vi "Insert Front Panel.vi"(8 "error in (no error)":errorcluster, 9 "Insertion Request Time":timestamp, 10 "Protected Subpanel":T1, 11 "IViewable in":refnum<class "IViewable.lvclass">) -> (0 "error out":errorcluster, 3 "IViewable out":refnum<class "IViewable.lvclass">)   [LabVIEW 2015, in "IViewable.lvlib" / "IViewable.lvclass"]
doc: "<License>\nCopyright © 2017 Composed Systems, LLC | All rights reserved\nwww.composed.io\n\nAuthor: Ethan Stern <ethan.stern@composed.io>\n\nThis software is provided \"AS IS\" WITHOUT WARRANTIES, either express or implied, AND IS FOR EDUCATIONAL PURPOSES ONLY.\n</License>"
uses:
  IViewable.lvclass
  ProtectedSubpanel/Protected Subpanel Reference.ctl
  ProtectedSubpanel/ProtectedSubpanel.lvclass
  IViewable.lvclass/IViewable.ctl
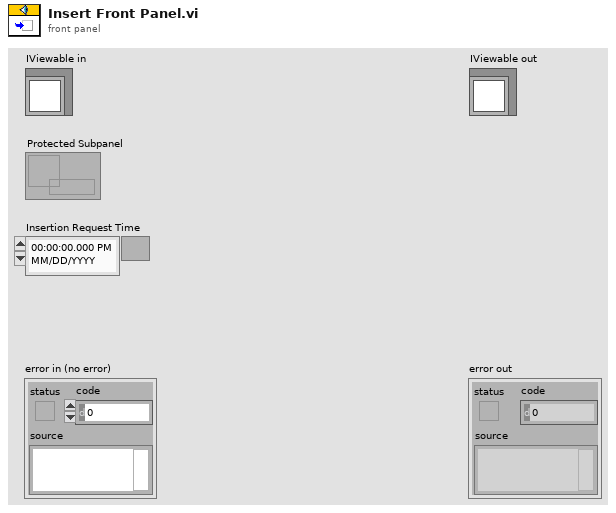
[diagram p1: front panel]
types:
  T1 = typedef "IViewable.lvlib/ProtectedSubpanel.lvclass/Protected Subpanel Reference.ctl" = refnum<data-value>
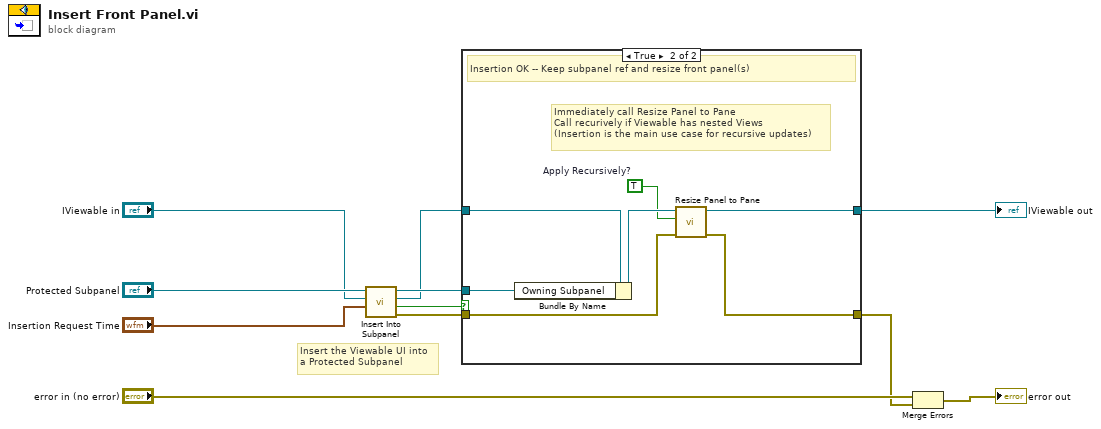
[diagram p0: block diagram]
diagram:
  # "Insert the Viewable UI into\na Protected Subpanel"
  n1 = call "Insert Into Subpanel.vi"("Insertion Request Time"="Insertion Request Time", "Viewable"="IViewable in", "Protected Subpanel"="Protected Subpanel") -> ("error out"=w6:errorcluster, "Inserted?"=w4:bool, "Viewable Out"=w1:refnum<class "IViewable.lvclass">, "Protected Subpanel"=w3:T1)  [unwired: 5 in]
  n2 = case shown="True" w4 {
    tunnel: w1 -> [w13 w20]
    tunnel: [w13 w19] -> w7
    tunnel: w6 -> [w12 w18]
    tunnel: w3 -> [_ w17]
    tunnel: [w12 w16] -> w5
    frame False {
      # "Insertion rejected or failed -- no additional action"
    }
    frame True {
      w14 = TRUE  # Apply Recursively?
      # "Immediately call Resize Panel to Pane\nCall recurively if Viewable has nested Views\n(Insertion is the main use case for recursive updates)"
      # "Insertion OK -- Keep subpanel ref and resize front panel(s)"
      n3 = Bundle By Name(cluster=w20, "Owning Subpanel"=w17) -> (w15:refnum<class "IViewable.lvclass">)
      n4 = call-dynamic "Resize Panel to Pane.vi"("error in (no error)"=w18, "Apply Recursively? (F)"=w14, "IViewable In"=w15) -> ("error out"=w16:errorcluster, "IViewable Out"=w19:refnum<class "IViewable.lvclass">)  [unwired: 7 in]
    }
  }
  "IViewable out" <- w7
  n5 = Merge Errors("error in (no error)", w5) -> (→"error out":errorcluster)
